vi "CALC_MARK_COUP_STAT_ON_OFF.vi"(0 "VISA IN":refnum<visa-resource-name>, 1 "Marker number":i32, 2 "Coupled Markers ON/OFF":bool, 5 "error in":errorcluster, 7 "Channel":i32) -> (14 "VISA Out":refnum<visa-resource-name>, 19 "error out":errorcluster)   [LabVIEW 2018, in "PNA-X.lvlib"]
doc: "CALCulate<cnum>:MARKer<mkr>:COUPling[:STATe]<ON|OFF> \n(Read-Write) Sets and Reads the state of Coupled Markers (ON and OFF) \nSee Critical Note \nParameters \n<cnum> Channel number of the measurement. There must be a selected measurement \non that channel. If unspecified, <cnum> is set to 1. \n<mkr> Any existing marker number from 1 to 10; if unspecified, value is set to 1. \n<ON|OFF> False (0) - Turns Coupled Markers OFF \nTrue (1) - Turns Coupled Markers ON \nExamples CALC:MARK:COUP ON \ncalculate2:marker8:coupling off \nQuery Syntax CALCulate<cnum>:MARKer<mkr>:COUPling:[STATe]? \nReturn Type Boolean (1 = ON, 0 = OFF) \nDefault OFF"
uses:
  PNA-X.lvlib
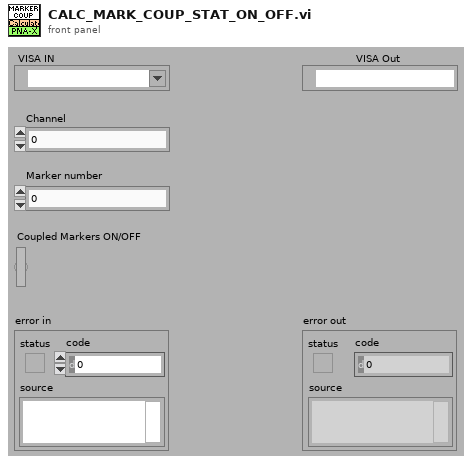
[diagram p1: front panel]
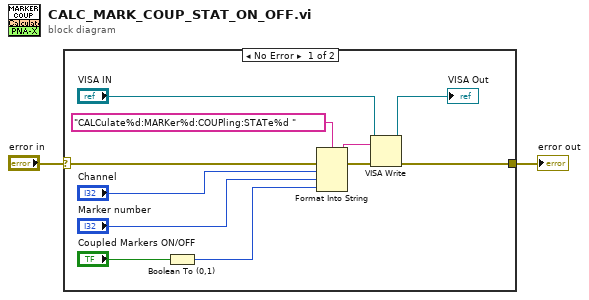
[diagram p0: block diagram]
diagram:
  n1 = case shown="No Error" "error in" {
    selector: "error in" -> [w13 w14]
    tunnel: [w8 w14] -> w1
    frame No Error {
      n2 = Boolean To (0,1)(Boolean="Coupled Markers ON/OFF") -> (0, 1=w3:i16)
      n3 = Format Into String(format string="CALCulate%d:MARKer%d:COUPling:STATe%d " ("Cmdline"), error in=w13, "Channel", "Marker number", w3) -> (resulting string=w11:string, error out=w12:errorcluster)  [unwired: 1 in]
      n4 = VISA Write(VISA resource name="VISA IN", write buffer=w11, error in (no error)=w12) -> (VISA resource name out=→"VISA Out":refnum<visa-resource-name>, error out=w8:errorcluster)  [unwired: 1 out]
    }
    frame Error {
    }
  }
  "error out" <- w1
